vi "pl1000Stop.vi"(8 "error in (no error)":errorcluster, 11 "pl1000 handle":i16) -> (0 "error out":errorcluster, 3 "pl1000 handle out":i16)   [LabVIEW 2010]
doc: "This function aborts data collection."
uses:
  pl1000.dll
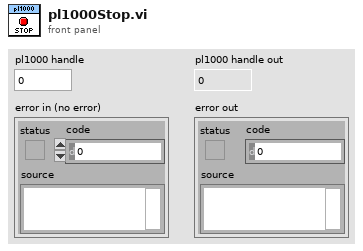
[diagram p1: front panel]
types:
  T1 = cluster{"status":bool, "code":u32, "source":string}
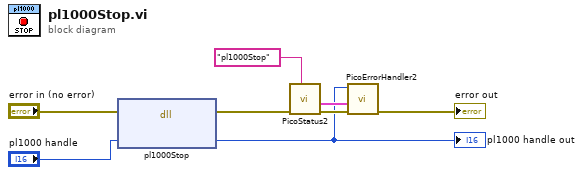
[diagram p0: block diagram]
diagram:
  n1 = dll-call lib="pl1000.dll" fn="pl1000Stop"(error in="error in (no error)", "handle"="pl1000 handle") -> (error out=w3:errorcluster, "handle"=w2:i16)  [unwired: 3 in, 1 out]
  "pl1000 handle out" <- w2
  n2 = call "PicoStatus2.vi"("PICO source"="pl1000Stop", "Error in"=w3) -> ("error out"=w6:errorcluster, "PICO_STATUS out"=w5:T1)  [unwired: 6 in]
  n3 = call "PicoErrorHandler2.vi"("error in (no error)"=w6, "PICO_STATUS in"=w5, "handle In"=w2) -> ("error out"=→"error out":errorcluster)  [unwired: 8 in]
